vi "Create.vi"(8 "error in":errorcluster, 9 "reset device":bool=TRUE, 10 "simulate":bool, 11 "topology name":T1="Configured Topology") -> (0 "error out":errorcluster, 3 "session factory out":refnum<class "Session Factory.lvclass">)   [LabVIEW 2021, in "Session Management niSwitch.lvlib" / "Session Factory.lvclass"]
uses:
  Session Factory.lvclass
  <instrlib>/niSwitch/niSwitch.llb/niSwitch Topologies.ctl
  Session Factory.lvclass/Session Factory.ctl
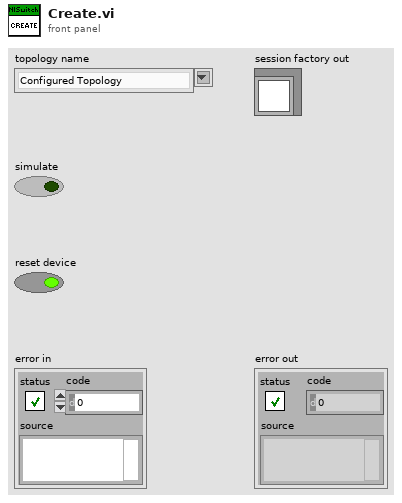
[diagram p1: front panel]
types:
  T1 = typedef "niSwitch Topologies.ctl" = string
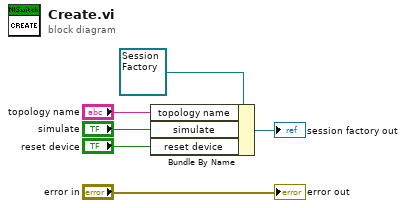
[diagram p0: block diagram]
diagram:
  n1 = Bundle By Name(cluster=refnum<class "Session Factory.lvclass"> refnum ("NI Session Management niSwitch.lvlib:Session Factory.lvclass"), "topology name"="topology name", "simulate"="simulate", "reset device"="reset device") -> (→"session factory out":refnum<class "Session Factory.lvclass">)
  "error out" <- "error in"
